vi "eFGV - Load New Config.vi"(6 "eFGV States":T1, 8 "Error In":errorcluster, 11 "Config from File":bool) -> (0 "Error Out":errorcluster, 2 "Event Config from File":refnum<user-event>)   [LabVIEW 2020]
uses:
  Control/State - eFGV.ctl
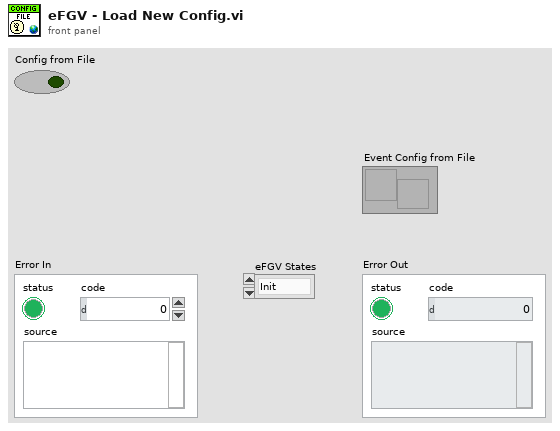
[diagram p1: front panel]
types:
  T1 = typedef "State - eFGV.ctl" = enum16{"Init", "Read", "Write", "Exit"}
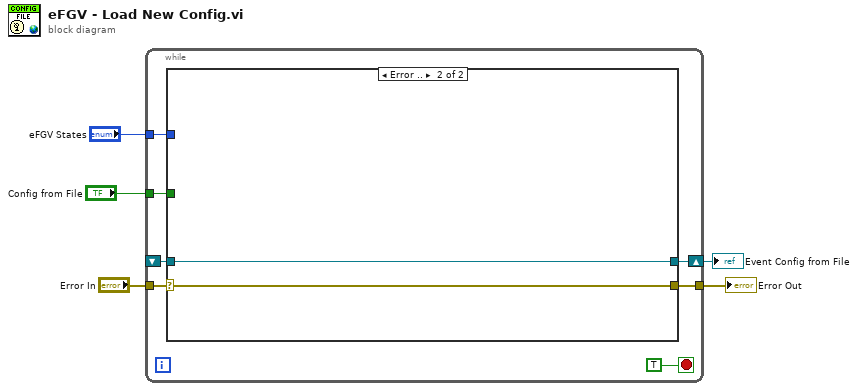
[diagram p0: block diagram]
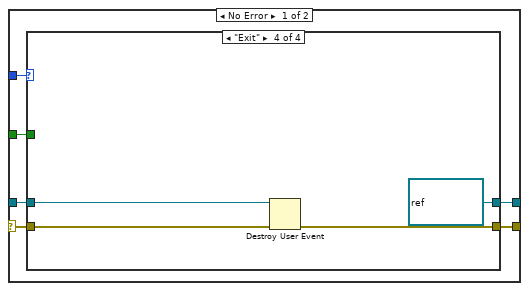
[diagram p2: hidden frame]
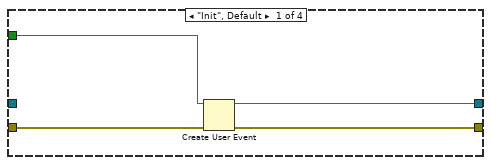
[diagram p3: hidden frame]
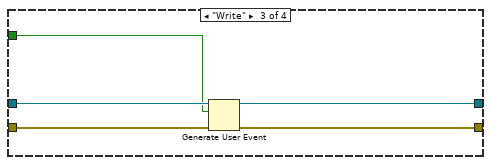
[diagram p5: hidden frame]
diagram:
  n1 = while {
    tunnel: "Error In" -> [w12]
    tunnel: [w11] -> w4
    tunnel: "eFGV States" -> [w9]
    tunnel: "Config from File" -> [w8]
    shift-right: [w7] -> w1
    shift-left: _ -> [w6]
    stop <- TRUE stop-if-true
    n2 = case shown="Error .." w12 {
      selector: w12 -> [w18 w35]
      tunnel: [w17 w35] -> w11
      tunnel: w9 -> [w16 _]
      tunnel: w8 -> [w15 _]
      tunnel: [w14 w34] -> w7
      tunnel: w6 -> [w13 w34]
      frame No Error {
        n3 = case shown="\"Exit\"" w16 {
          tunnel: w18 -> [w22 w24 w29 w33]
          tunnel: [w21 w24 w28 w32] -> w17
          tunnel: w15 -> [w20 _ w25 _]
          tunnel: [w19 w23 w26 refnum<user-event> refnum ("Config from File")] -> w14
          tunnel: w13 -> [_ w23 w27 w31]
          frame "Init", Default {
            n4 = Create User Event(user event datatype=w20, error in=w22) -> (user event=w19:refnum<user-event>, error out=w21:errorcluster)
          }
          frame "Read" {
          }
          frame "Write" {
            n5 = Generate User Event(user event=w27, event data cluster=w25, error in=w29) -> (user event out=w26:refnum<user-event>, error out=w28:errorcluster)  [unwired: 1 in]
          }
          frame "Exit" {
            n6 = Destroy User Event(user event=w31, error in=w33) -> (error out=w32:errorcluster)
          }
        }
      }
      frame Error {
      }
    }
  }
  "Error Out" <- w4
  "Event Config from File" <- w1
